vi "初始化.vi"(8 "错误输入（无错误）":errorcluster, 11 "引用输入":refnum<vi>) -> (0 "错误输出":errorcluster, 3 "引用输出":refnum<vi>)   [LabVIEW 8.6, in "窗口操作.lvlib"]
doc: "<B>引用输入：</B>需要改变窗口的引用\n<B>引用输出：</B>需要改变窗口的引用输出\n\n编写者 ：曾嘉康\n编写时间：2014/12/12"
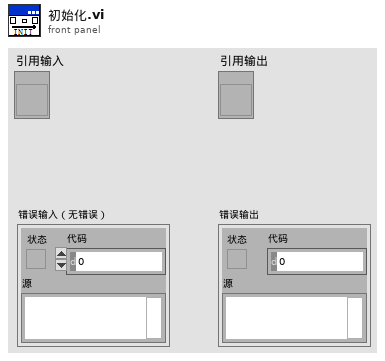
[diagram p1: front panel]
types:
  T1 = enum32{"Invalid", "Standard", "Closed", "Hidden", "Minimized", "Maximized"}
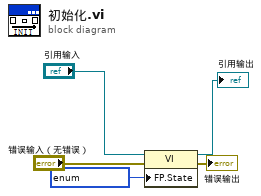
[diagram p0: block diagram]
diagram:
  n1 = property class="VI"(reference="引用输入", error in="错误输入（无错误）", "FP.State"=T1 ? ("前面板窗口:状态")) -> (reference out=→"引用输出":refnum<vi>, error out=→"错误输出":errorcluster)
